vi "Python@File(Worker)__Parameter.vi"(1 "ParamterIn":string) -> (0 "ParamterOut":string)   [LabVIEW 2020]
uses:
  MainFrame/Global.vi
panel:
  in  "Session":string(combo)
  in  "FileName":string(combo)
  in  "Confirm":bool
  # "Python@File(Worker) $Worker,$PythonFile"
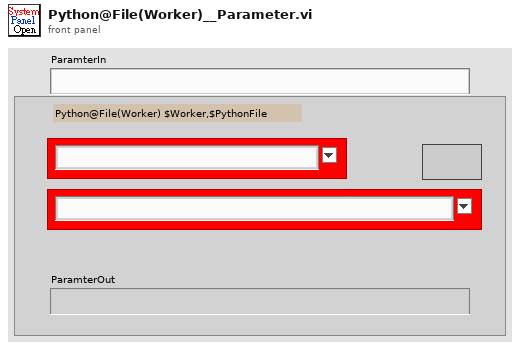
[diagram p1: front panel]
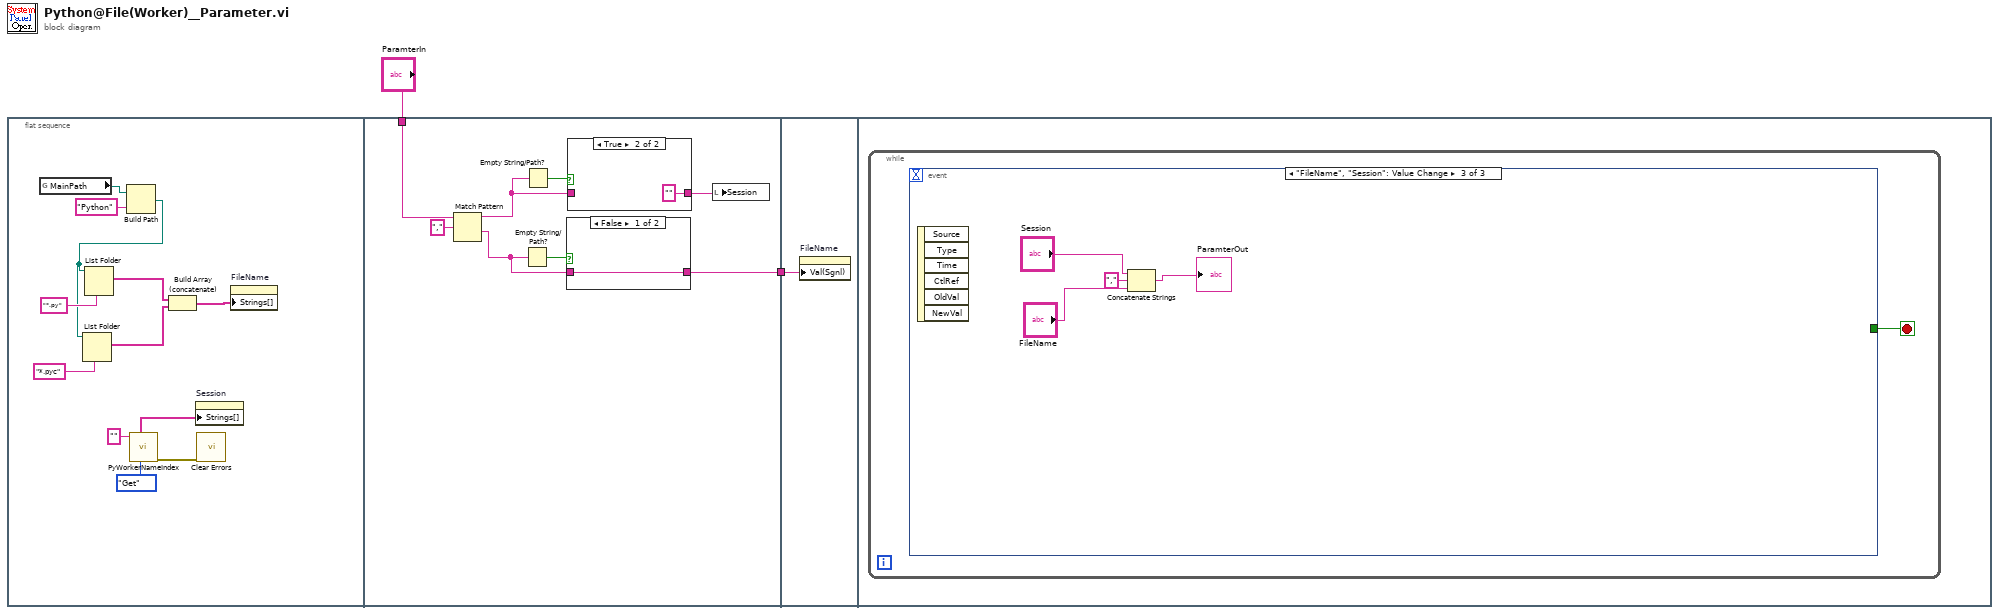
[diagram p0: block diagram]
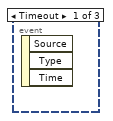
[diagram p4: hidden frame]
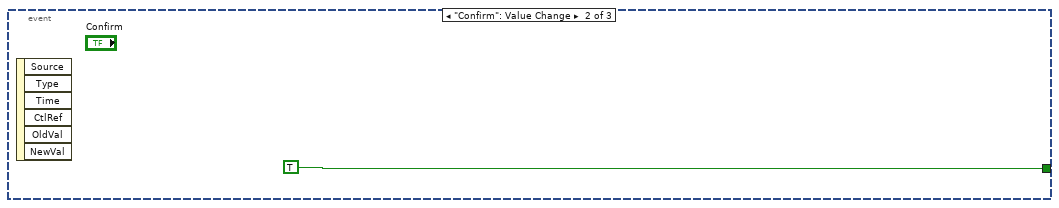
[diagram p5: hidden frame]
diagram:
  n1 = flat-sequence {
    tunnel: "ParamterIn" -> [w20]
    tunnel: [w21] -> w1
    tunnel: w1 -> [w27]
    frame #0 {
      n2 = global read "Global.vi" "MainPath"() -> (w13:path)
      n3 = Build Path(base path=w13, name or relative path="Python") -> (appended path=w10:path)
      n4 = List Folder(path=w10, pattern="*.pyc") -> (filenames=w8:string[])  [unwired: 2 in, 3 out]
      n5 = List Folder(path=w10, pattern="*.py") -> (filenames=w9:string[])  [unwired: 2 in, 3 out]
      n6 = call "PyWorkerNameIndex.vi"("OP"=enum16{"Init", "Get", "Set"}."Get", "WrokerName"="" ("SessionIn")) -> ("error out"=w3:errorcluster, "PythonWorkerNameS"=w4:string[])  [unwired: 6 in, 2 out]
      n7 = Build Array (concatenate)(w9, w8) -> (w7:string[])
      n8 = property on="Session" class="CmbBox"("Strings[]"=w4) -> ()  [unwired: 2 in, 2 out]
      n9 = call <vilib>:"Clear Errors.vi"("error in (no error)"=w3) -> ()  [unwired: 5 in, 2 out]
      n10 = property on="FileName" class="CmbBox"("Strings[]"=w7) -> ()  [unwired: 2 in, 2 out]
    }
    frame #1 {
      n11 = Match Pattern(string=w20, regular expression=",") -> (before substring=w16:string, after substring=w18:string)  [unwired: 1 in, 2 out]
      n12 = Empty String/Path?(string/path=w18) -> (empty?=w22:bool)
      n13 = Empty String/Path?(string/path=w16) -> (empty?=w17:bool)
      n14 = case shown="False" w22 {
        tunnel: w18 -> [w25 w26]
        tunnel: [w25 w26] -> w21
        frame False {
        }
        frame True {
        }
      }
      n15 = case shown="True" w17 {
        tunnel: w16 -> [w23 _]
        tunnel: [w23 "" ("ParamterIn")] -> w15
        frame False {
        }
        frame True {
        }
      }
      n16 = local write "Session"(w15) -> ()
    }
    frame #2 {
      n17 = property on="FileName" class="CmbBox"("Val(Sgnl)"=w27) -> ()  [unwired: 2 in, 2 out]
    }
    frame #3 {
      n18 = while {
        stop <- w28 stop-if-true
        n19 = event shown="[2] \"FileName\", \"Session\": Value Change" {
          selector: _ -> [_ _ _]
          dyn-events: _ -> [_ _ _]
          timeout: _ -> [_ _ _]
          tunnel: [_ TRUE _] -> w28
          event Timeout {
            n20 = event-data() -> ()  [unwired: 1 in, 3 out]
          }
          event "Confirm": Value Change {
            n21 = event-data() -> ()  [unwired: 1 in, 6 out]
          }
          event "FileName", "Session": Value Change {
            n22 = event-data() -> ()  [unwired: 1 in, 6 out]
            n23 = Concatenate Strings("Session", "," ("string"), "FileName") -> (→"ParamterOut":string)
          }
        }
      }
    }
  }
